vi "VDI Read Bytes.vi"(4 "AftClkCnt":u16, 5 "PreClkCnt":u16, 6 "ReadLen":u8, 7 "Addr":u8, 9 "Channel":u8, 10 "DevIndex":i32, 11 "DevType":i32) -> (2 "function return":i32, 3 "pReadData":u8[](array[numeric]))   [LabVIEW 2010, in "ControlDigRF.lvlib"]
doc: "int WINAPI VDI_ReadBytes(int DevType,int DevIndex,unsigned char Channel,unsigned char Addr,unsigned char *pReadData,unsigned char ReadLen,unsigned short PreClkCnt,unsigned short AftClkCnt);"
uses:
  ControlDigRF.lvlib
  ControlDigRF/Ginkgo_Driver.dll
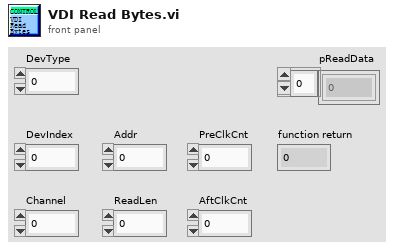
[diagram p1: front panel]
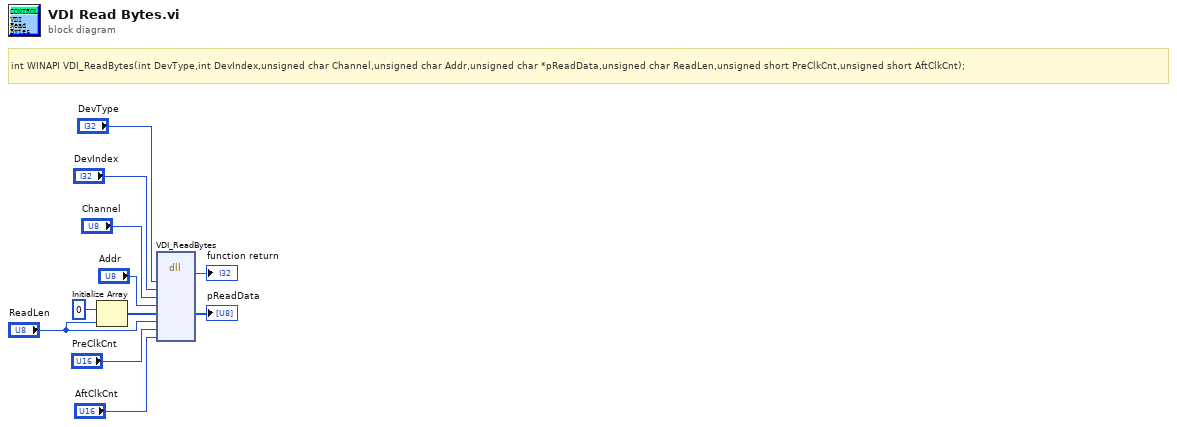
[diagram p0: block diagram]
diagram:
  # "int WINAPI VDI_ReadBytes(int DevType,int DevIndex,unsigned char Channel,unsigned char Addr,unsigned char *pReadData,unsigned char ReadLen,unsigned short PreClkCnt,unsigned short AftClkCnt);"
  n1 = Initialize Array(u8 0 ("element"), "ReadLen") -> (w6:u8[])
  n2 = dll-call lib="E:/Project/vt_ginkgo/truck/Ginkgo Driver/vs2010/Ginkgo_USB-I2C&SPI&CAN_API_v2.0.3.3/lib/labview_32bit/ControlDigRF/Ginkgo_Driver.*" fn="VDI_ReadBytes"("DevType"="DevType", "DevIndex"="DevIndex", "Channel"="Channel", "Addr"="Addr", "pReadData"=w6, "ReadLen"="ReadLen", "PreClkCnt"="PreClkCnt", "AftClkCnt"="AftClkCnt") -> (→"function return":i32, "pReadData"=→"pReadData":u8[])  [unwired: 10 in, 2 out]
